vi "ConvertPressureToPercent.vi"(10 "Pressure Setpoint":dbl, 11 "Full Scale (bar a)":dbl) -> (3 "% of full scale":sgl)   [LabVIEW 2019]
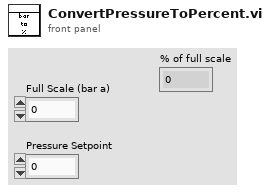
[diagram p1: front panel]
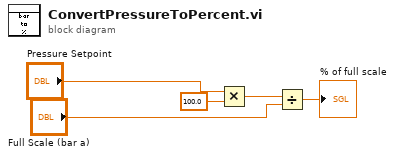
[diagram p0: block diagram]
diagram:
  n1 = Multiply(x="Pressure Setpoint", y=100.0) -> (x*y=w4:dbl)
  n2 = Divide(x=w4, y="Full Scale (bar a)") -> (x/y=→"% of full scale":dbl)
